vi "Test_ExplicitlyNamedI32_ValueOK.vi"(8 "error in (no error)":errorcluster, 11 "TestCase in":refnum<class "TestCurrentValueTable.lvclass">) -> (0 "error out":errorcluster, 3 "TestCase out":refnum<class "TestCurrentValueTable.lvclass">)   [LabVIEW 2015, in "CurrentValueTable.lvlib" / "TestCurrentValueTable.lvclass"]
uses:
  TestCurrentValueTable.lvclass
  <vilib>/addons/_JKI Toolkits/VI Tester/TestCase.llb/TestCase.lvclass
  CurrentValueTable.lvclass
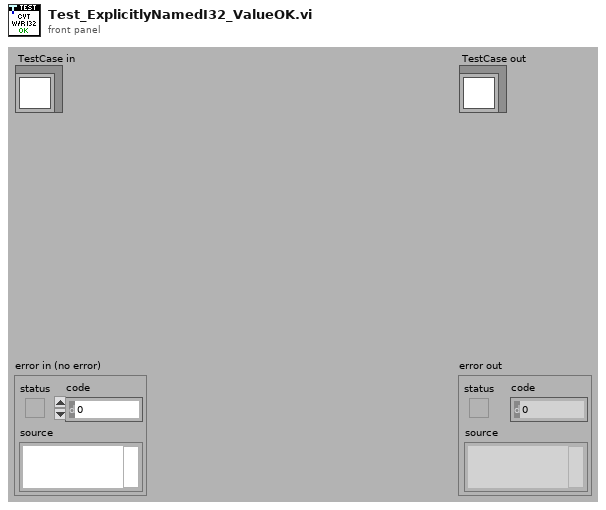
[diagram p1: front panel]
types:
  T1 = typedef "CurrentValueTable.lvlib/CurrentValueTable.lvclass/CurrentValueTable Reference.ctl" = refnum<data-value>
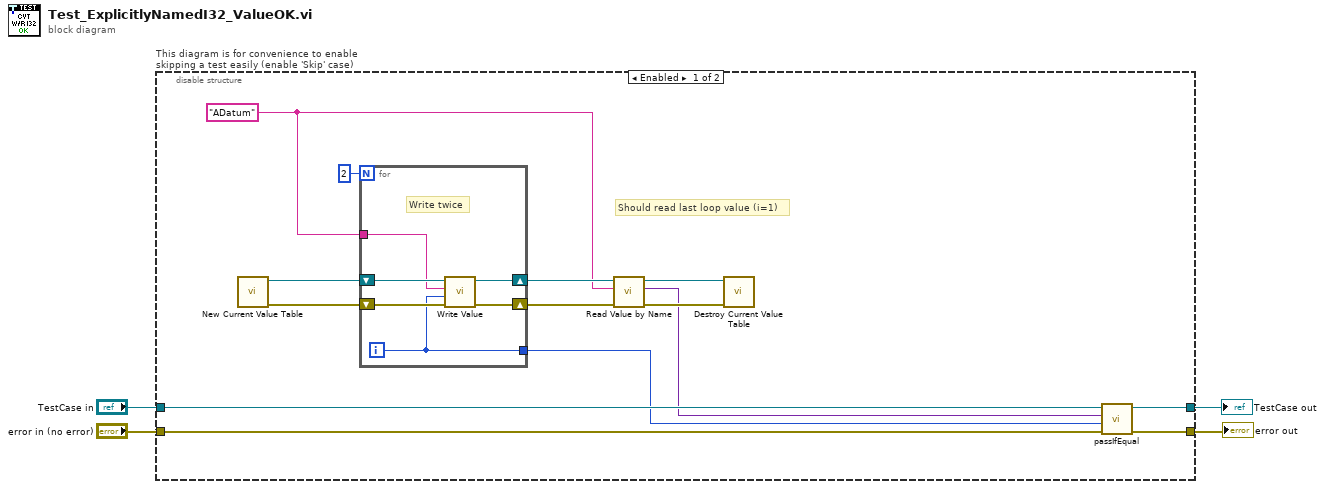
[diagram p0: block diagram]
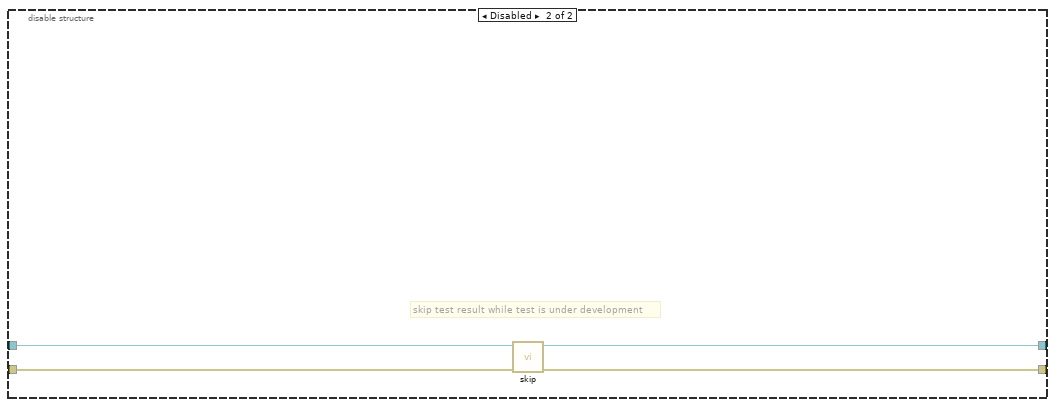
[diagram p2: hidden frame]
diagram:
  n1 = disable-structure "This diagram is for convenience to enable skipping a test easily (enable 'Skip' case)" shown="Enabled" {
    disable-tunnel: "TestCase in" -> [w18 w28]
    disable-tunnel: [w17 w26] -> w1
    disable-tunnel: [w16 w27] -> w3
    disable-tunnel: "error in (no error)" -> [w15 w25]
    frame Enabled {
      w7 = "ADatum" ("Data Name (Use Value Name)")
      # "Should read last loop value (i=1)"
      n2 = call "New Current Value Table.vi"() -> ("error out"=w12:errorcluster, "Current Value Table"=w14:T1)  [unwired: 10 in]
      n3 = for {
        N: 2 -> [_]
        shift-right: [w23] -> w13
        shift-left: w14 -> [w24]
        shift-right: [w21] -> w9
        shift-left: w12 -> [w22]
        tunnel: w7 -> [w20]
        tunnel: [w19] -> w5
        i -> [w19]
        # "Write twice"
        n4 = call "Write Value.vi"("error in (no error)"=w22, "Value"=w19, "Data Name (Use Value Name)"=w20, "Current Value Table"=w24) -> ("error out"=w21:errorcluster, "Current Value Table"=w23:T1)  [unwired: 6 in]
      }
      n5 = call "Read Value by Name.vi"("error in (no error)"=w9, "Data Name"=w7, "Current Value Table"=w13) -> ("error out"=w8:errorcluster, "Current Value"=w6:variant, "Current Value Table"=w10:T1)  [unwired: 5 in, 1 out]
      n6 = call "Destroy Current Value Table.vi"("error in (no error)"=w8, "Current Value Table"=w10) -> ()  [unwired: 9 in, 1 out]
      n7 = call-dynamic "passIfEqual.vi"("error in (no error)"=w15, "y"=w5, "x"=w6, "TestCase in"=w18) -> ("error out"=w16:errorcluster, "TestCase out"=w17:refnum<class "TestCurrentValueTable.lvclass">)  [unwired: 6 in]
    }
    frame Disabled {
      # "skip test result while test is under development"
      n8 = call <vilib>:"skip.vi"("error in (no error)"=w25, "TestCase in"=w28) -> ("error out"=w27:errorcluster, "TestCase out"=w26:refnum<class "TestCurrentValueTable.lvclass">)  [unwired: 8 in]
    }
  }
  "error out" <- w3
  "TestCase out" <- w1
